vi "ex7.vi"() -> ()   [LabVIEW 2022 SP3]
panel:
  in  "C":bool
  in  "B":bool
  in  "A":bool
  out "Result: True?":bool
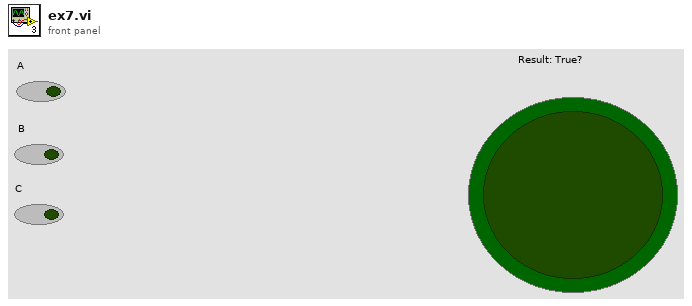
[diagram p1: front panel]
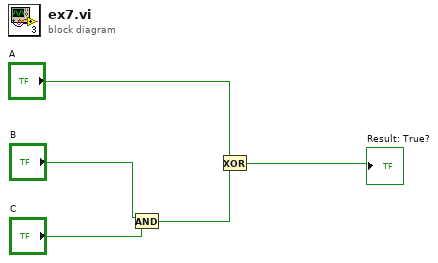
[diagram p0: block diagram]
diagram:
  n1 = And(x="B", y="C") -> (x .and. y?=w2:bool)
  n2 = Exclusive Or(1:w2, 2:"A") -> (0:→"Result: True?":bool)
